vi "material_parameter_strings_to_strict_type.vi"(8 "error in (no error)":errorcluster, 10 "Material parameters (strings)":T2) -> (0 "error out":errorcluster, 2 "Material parameters":T1)   [LabVIEW 2018]
uses:
  material_parameters_strings.ctl
  material_parameters.ctl
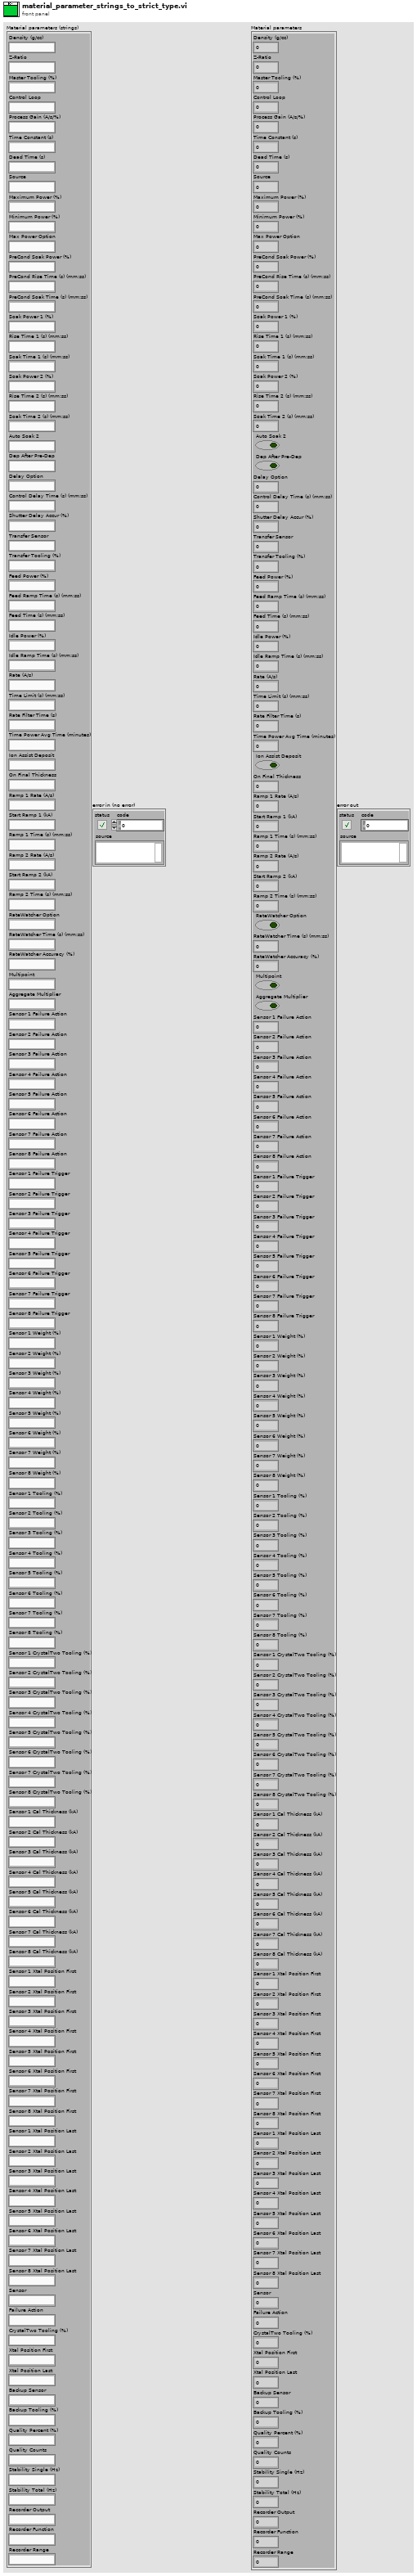
[diagram p1: front panel]
types:
  T1 = typedef "material_parameters.ctl" = cluster{"Density (g/cc)":sgl, "Z-Ratio":sgl, "Master Tooling (%)":sgl, "Control Loop":u8, "Process Gain (A/s/%)":sgl, "Time Constant (s)":sgl, "Dead Time (s)":sgl, "Source":u8, "Maximum Power (%)":sgl, "Minimum Power (%)":sgl, "Max Power Option":u8, "PreCond Soak Power (%)":sgl, "PreCond Rise Time (s) (mm:ss)":u16, "PreCond Soak Time (s) (mm:ss)":u16, "Soak Power 1 (%)":sgl, "Rise Time 1 (s) (mm:ss)":u16, "Soak Time 1 (s) (mm:ss)":u16, "Soak Power 2 (%)":sgl, "Rise Time 2 (s) (mm:ss)":u16, "Soak Time 2 (s) (mm:ss)":u16, "Auto Soak 2":bool, "Dep After Pre-Dep":bool, "Delay Option":u8, "Control Delay Time (s) (mm:ss)":u16, "Shutter Delay Accur (%)":u8, "Transfer Sensor":u8, "Transfer Tooling (%)":sgl, "Feed Power (%)":sgl, "Feed Ramp Time (s) (mm:ss)":u16, "Feed Time (s) (mm:ss)":u16, "Idle Power (%)":sgl, "Idle Ramp Time (s) (mm:ss)":u16, "Rate (A/s)":sgl, "Time Limit (s) (mm:ss)":u16, "Rate Filter Time (s)":u8, "Time Power Avg Time (minutes)":u8, "Ion Assist Deposit":bool, "On Final Thickness":u8, "Ramp 1 Rate (A/s)":sgl, "Start Ramp 1 (kA)":sgl, "Ramp 1 Time (s) (mm:ss)":u16, "Ramp 2 Rate (A/s)":sgl, "Start Ramp 2 (kA)":sgl, "Ramp 2 Time (s) (mm:ss)":u16, "RateWatcher Option":bool, "RateWatcher Time (s) (mm:ss)":u16, "RateWatcher Accuracy (%)":u8, "Multipoint":bool, "Aggregate Multiplier":bool, "Sensor 1 Failure Action":u8, "Sensor 2 Failure Action":u8, "Sensor 3 Failure Action":u8, "Sensor 4 Failure Action":u8, "Sensor 5 Failure Action":u8, "Sensor 6 Failure Action":u8, "Sensor 7 Failure Action":u8, "Sensor 8 Failure Action":u8, "Sensor 1 Failure Trigger":u8, "Sensor 2 Failure Trigger":u8, "Sensor 3 Failure Trigger":u8, "Sensor 4 Failure Trigger":u8, "Sensor 5 Failure Trigger":u8, "Sensor 6 Failure Trigger":u8, "Sensor 7 Failure Trigger":u8, "Sensor 8 Failure Trigger":u8, "Sensor 1 Weight (%)":sgl, "Sensor 2 Weight (%)":sgl, "Sensor 3 Weight (%)":sgl, "Sensor 4 Weight (%)":sgl, "Sensor 5 Weight (%)":sgl, "Sensor 6 Weight (%)":sgl, "Sensor 7 Weight (%)":sgl, "Sensor 8 Weight (%)":sgl, "Sensor 1 Tooling (%)":sgl, "Sensor 2 Tooling (%)":sgl, "Sensor 3 Tooling (%)":sgl, "Sensor 4 Tooling (%)":sgl, "Sensor 5 Tooling (%)":sgl, "Sensor 6 Tooling (%)":sgl, "Sensor 7 Tooling (%)":sgl, "Sensor 8 Tooling (%)":sgl, "Sensor 1 CrystalTwo Tooling (%)":sgl, "Sensor 2 CrystalTwo Tooling (%)":sgl, "Sensor 3 CrystalTwo Tooling (%)":sgl, "Sensor 4 CrystalTwo Tooling (%)":sgl, "Sensor 5 CrystalTwo Tooling (%)":sgl, "Sensor 6 CrystalTwo Tooling (%)":sgl, "Sensor 7 CrystalTwo Tooling (%)":sgl, "Sensor 8 CrystalTwo Tooling (%)":sgl, "Sensor 1 Cal Thickness (kA)":sgl, "Sensor 2 Cal Thickness (kA)":sgl, "Sensor 3 Cal Thickness (kA)":sgl, "Sensor 4 Cal Thickness (kA)":sgl, "Sensor 5 Cal Thickness (kA)":sgl, "Sensor 6 Cal Thickness (kA)":sgl, "Sensor 7 Cal Thickness (kA)":sgl, "Sensor 8 Cal Thickness (kA)":sgl, "Sensor 1 Xtal Position First":u8, "Sensor 2 Xtal Position First":u8, "Sensor 3 Xtal Position First":u8, "Sensor 4 Xtal Position First":u8, "Sensor 5 Xtal Position First":u8, "Sensor 6 Xtal Position First":u8, "Sensor 7 Xtal Position First":u8, "Sensor 8 Xtal Position First":u8, "Sensor 1 Xtal Position Last":u8, "Sensor 2 Xtal Position Last":u8, "Sensor 3 Xtal Position Last":u8, "Sensor 4 Xtal Position Last":u8, "Sensor 5 Xtal Position Last":u8, "Sensor 6 Xtal Position Last":u8, "Sensor 7 Xtal Position Last":u8, "Sensor 8 Xtal Position Last":u8, "Sensor":u8, "Failure Action":u8, "CrystalTwo Tooling (%)":sgl, "Xtal Position First":u8, "Xtal Position Last":u8, "Backup Sensor":u8, "Backup Tooling (%)":sgl, "Quality Percent (%)":u8, "Quality Counts":u8, "Stability Single (Hz)":u8, "Stability Total (Hz)":u8, "Recorder Output":u8, "Recorder Function":u8, "Recorder Range":u8}
  T2 = typedef "material_parameters_strings.ctl" = cluster{"Density (g/cc)":string, "Z-Ratio":string, "Master Tooling (%)":string, "Control Loop":string, "Process Gain (A/s/%)":string, "Time Constant (s)":string, "Dead Time (s)":string, "Source":string, "Maximum Power (%)":string, "Minimum Power (%)":string, "Max Power Option":string, "PreCond Soak Power (%)":string, "PreCond Rise Time (s) (mm:ss)":string, "PreCond Soak Time (s) (mm:ss)":string, "Soak Power 1 (%)":string, "Rise Time 1 (s) (mm:ss)":string, "Soak Time 1 (s) (mm:ss)":string, "Soak Power 2 (%)":string, "Rise Time 2 (s) (mm:ss)":string, "Soak Time 2 (s) (mm:ss)":string, "Auto Soak 2":string, "Dep After Pre-Dep":string, "Delay Option":string, "Control Delay Time (s) (mm:ss)":string, "Shutter Delay Accur (%)":string, "Transfer Sensor":string, "Transfer Tooling (%)":string, "Feed Power (%)":string, "Feed Ramp Time (s) (mm:ss)":string, "Feed Time (s) (mm:ss)":string, "Idle Power (%)":string, "Idle Ramp Time (s) (mm:ss)":string, "Rate (A/s)":string, "Time Limit (s) (mm:ss)":string, "Rate Filter Time (s)":string, "Time Power Avg Time (minutes)":string, "Ion Assist Deposit":string, "On Final Thickness":string, "Ramp 1 Rate (A/s)":string, "Start Ramp 1 (kA)":string, "Ramp 1 Time (s) (mm:ss)":string, "Ramp 2 Rate (A/s)":string, "Start Ramp 2 (kA)":string, "Ramp 2 Time (s) (mm:ss)":string, "RateWatcher Option":string, "RateWatcher Time (s) (mm:ss)":string, "RateWatcher Accuracy (%)":string, "Multipoint":string, "Aggregate Multiplier":string, "Sensor 1 Failure Action":string, "Sensor 2 Failure Action":string, "Sensor 3 Failure Action":string, "Sensor 4 Failure Action":string, "Sensor 5 Failure Action":string, "Sensor 6 Failure Action":string, "Sensor 7 Failure Action":string, "Sensor 8 Failure Action":string, "Sensor 1 Failure Trigger":string, "Sensor 2 Failure Trigger":string, "Sensor 3 Failure Trigger":string, "Sensor 4 Failure Trigger":string, "Sensor 5 Failure Trigger":string, "Sensor 6 Failure Trigger":string, "Sensor 7 Failure Trigger":string, "Sensor 8 Failure Trigger":string, "Sensor 1 Weight (%)":string, "Sensor 2 Weight (%)":string, "Sensor 3 Weight (%)":string, "Sensor 4 Weight (%)":string, "Sensor 5 Weight (%)":string, "Sensor 6 Weight (%)":string, "Sensor 7 Weight (%)":string, "Sensor 8 Weight (%)":string, "Sensor 1 Tooling (%)":string, "Sensor 2 Tooling (%)":string, "Sensor 3 Tooling (%)":string, "Sensor 4 Tooling (%)":string, "Sensor 5 Tooling (%)":string, "Sensor 6 Tooling (%)":string, "Sensor 7 Tooling (%)":string, "Sensor 8 Tooling (%)":string, "Sensor 1 CrystalTwo Tooling (%)":string, "Sensor 2 CrystalTwo Tooling (%)":string, "Sensor 3 CrystalTwo Tooling (%)":string, "Sensor 4 CrystalTwo Tooling (%)":string, "Sensor 5 CrystalTwo Tooling (%)":string, "Sensor 6 CrystalTwo Tooling (%)":string, "Sensor 7 CrystalTwo Tooling (%)":string, "Sensor 8 CrystalTwo Tooling (%)":string, "Sensor 1 Cal Thickness (kA)":string, "Sensor 2 Cal Thickness (kA)":string, "Sensor 3 Cal Thickness (kA)":string, "Sensor 4 Cal Thickness (kA)":string, "Sensor 5 Cal Thickness (kA)":string, "Sensor 6 Cal Thickness (kA)":string, "Sensor 7 Cal Thickness (kA)":string, "Sensor 8 Cal Thickness (kA)":string, "Sensor 1 Xtal Position First":string, "Sensor 2 Xtal Position First":string, "Sensor 3 Xtal Position First":string, "Sensor 4 Xtal Position First":string, "Sensor 5 Xtal Position First":string, "Sensor 6 Xtal Position First":string, "Sensor 7 Xtal Position First":string, "Sensor 8 Xtal Position First":string, "Sensor 1 Xtal Position Last":string, "Sensor 2 Xtal Position Last":string, "Sensor 3 Xtal Position Last":string, "Sensor 4 Xtal Position Last":string, "Sensor 5 Xtal Position Last":string, "Sensor 6 Xtal Position Last":string, "Sensor 7 Xtal Position Last":string, "Sensor 8 Xtal Position Last":string, "Sensor":string, "Failure Action":string, "CrystalTwo Tooling (%)":string, "Xtal Position First":string, "Xtal Position Last":string, "Backup Sensor":string, "Backup Tooling (%)":string, "Quality Percent (%)":string, "Quality Counts":string, "Stability Single (Hz)":string, "Stability Total (Hz)":string, "Recorder Output":string, "Recorder Function":string, "Recorder Range":string}
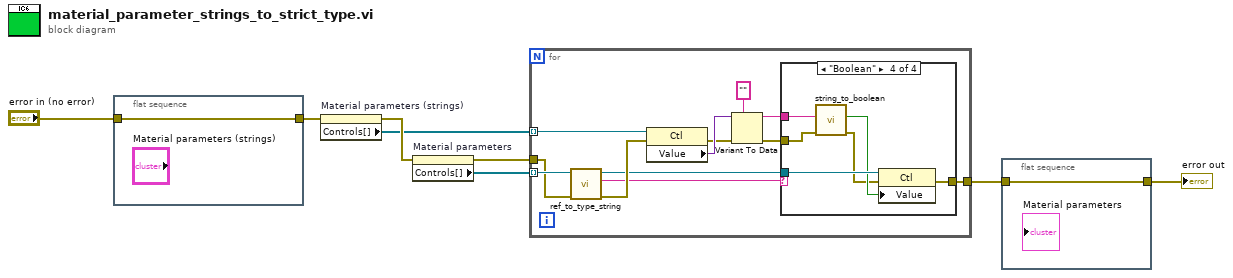
[diagram p0: block diagram]
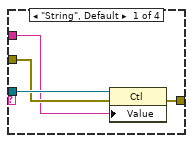
[diagram p2: hidden frame]
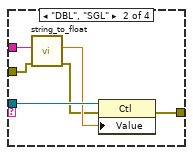
[diagram p3: hidden frame]
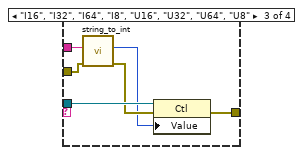
[diagram p4: hidden frame]
diagram:
  n1 = flat-sequence {
    tunnel: "error in (no error)" -> [w9]
    tunnel: [w9] -> w6
    frame #0 {
    }
  }
  n2 = property on="Material parameters (strings)" class="Clust (strict)"(error in=w6) -> (error out=w8:errorcluster, "Controls[]"=w2:refnum<vi>[])  [unwired: 1 in, 1 out]
  n3 = property on="Material parameters" class="Clust (strict)"(error in=w8) -> (error out=w4:errorcluster, "Controls[]"=w3:refnum<vi>[])  [unwired: 1 in, 1 out]
  n4 = for {
    tunnel: w2 -> [w21] mode=indexing
    tunnel: w3 -> [w14] mode=indexing
    tunnel: w4 -> [w13]
    tunnel: [w20] -> w1
    n5 = call "ref_to_type_string.vi"("error in (no error)"=w13, "Control ref in"=w14) -> ("error out"=w12:errorcluster, "Type String"=w10:string, "Control ref out"=w11:refnum<vi>)  [unwired: 7 in]
    n6 = property class="Ctl"(reference=w21, error in=w12) -> (error out=w17:errorcluster, "Value"=w18:variant)  [unwired: 1 out]
    n7 = Variant To Data(error in=w17, type="", Variant=w18) -> (data=w16:string, error out=w15:errorcluster)
    n8 = case shown="\"Boolean\"" w10 {
      tunnel: w11 -> [w25 w31 w37 w43]
      tunnel: [w24 w30 w36 w42] -> w20
      tunnel: w16 -> [w22 w29 w35 w38]
      tunnel: w15 -> [w23 w27 w34 w41]
      frame "String", Default {
        n9 = property class="Ctl"(reference=w25, error in=w23, "Value"=w22) -> (error out=w24:errorcluster)  [unwired: 1 out]
      }
      frame "DBL", "SGL" {
        n10 = call "string_to_float.vi"("error in (no error)"=w27, "Float (string)"=w29) -> ("error out"=w26:errorcluster, "Float (sgl)"=w28:sgl)  [unwired: 8 in]
        n11 = property class="Ctl"(reference=w31, error in=w26, "Value"=w28) -> (error out=w30:errorcluster)  [unwired: 1 out]
      }
      frame "I16", "I32", "I64", "I8", "U16", "U32", "U64", "U8" {
        n12 = call "string_to_int.vi"("error in (no error)"=w34, "Int (string)"=w35) -> ("error out"=w33:errorcluster, "Int"=w32:i32)  [unwired: 8 in]
        n13 = property class="Ctl"(reference=w37, error in=w33, "Value"=w32) -> (error out=w36:errorcluster)  [unwired: 1 out]
      }
      frame "Boolean" {
        n14 = call "string_to_boolean.vi"("error in (no error)"=w41, "Int (string)"=w38) -> ("error out"=w39:errorcluster, "Boolean"=w40:bool)  [unwired: 8 in]
        n15 = property class="Ctl"(reference=w43, error in=w39, "Value"=w40) -> (error out=w42:errorcluster)  [unwired: 1 out]
      }
    }
  }
  n16 = flat-sequence {
    tunnel: w1 -> [w44]
    tunnel: [w44] -> w5
    frame #0 {
    }
  }
  "error out" <- w5
